vi "Message_Update_Calib_frontpanel.vi"(8 "error in (no error)":errorcluster, 11 "Message":string) -> (0 "error out":errorcluster)   [LabVIEW 2020]
uses:
  Globals/gl_Calibration globals.vi
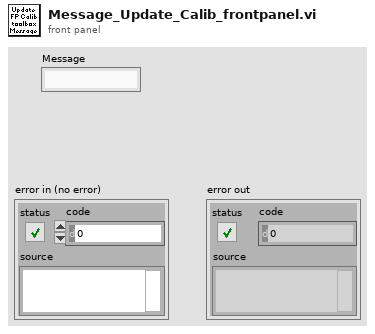
[diagram p1: front panel]
types:
  T1 = typedef "AOL Z cal process refs.ctl" = cluster{"This VI":refnum<vi>, "Abort (ind)":refnum<vi>, "Next (ind)":refnum<vi>, "Cancel":refnum<vi>, "Next":refnum<vi>, "Message":refnum<vi>, "Progress":refnum<vi>}
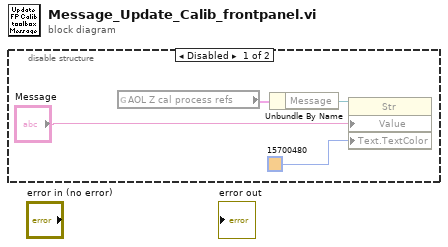
[diagram p0: block diagram]
diagram:
  n1 = disable-structure shown="Disabled" {
    frame Disabled {
      n2 = global read "gl_Calibration globals.vi" "AOL Z cal process refs"() -> (w2:T1)
      n3 = Unbundle By Name(w2) -> ("Message"=w3:refnum<vi>)
      n4 = property class="Str"(reference=w3, "Value"="Message", "Text.TextColor"=u32 15700480) -> ()  [unwired: 1 in, 2 out]
    }
    frame Enabled {
    }
  }
